vi "Query Multi Eval Meas Spectrum Limit Check Results.vi"(0 "VISA resource name":refnum<visa-resource-name>, 5 "Instance (1)":i32=1, 7 "Result Type (Current)":i32(ring) items=["Current"=0, "Maximum"=4], 11 "error in (no error)":errorcluster) -> (4 "VISA resource name out":refnum<visa-resource-name>, 6 "Reliability":i32, 8 "Limit Check Results":dbl[](array[numeric]), 14 "Out Of Tolerance":i32, 15 "error out":errorcluster)   [LabVIEW 2020, in "Rohde&Schwarz CMP LR WPAN Measurement.lvlib"]
doc: "Returns the spectrum limit check single results.\n\nAttribute:\n-\n\nRemote-control commands:\nCALCulate:WPAN:MEAS<i>:MEValuation:SPECtrum:CURRent?\nCALCulate:WPAN:MEAS<i>:MEValuation:SPECtrum:MAXimum?"
uses:
  <instrlib>/Rohde&Schwarz CMP LR WPAN Measurement/Rohde&Schwarz CMP LR WPAN Measurement.lvlib
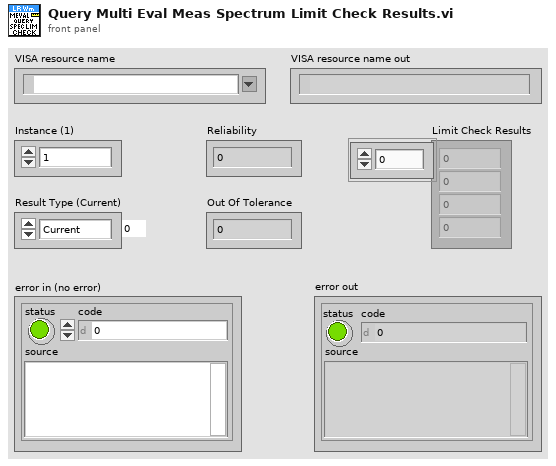
[diagram p1: front panel]
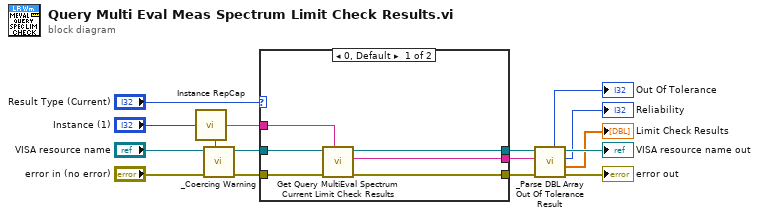
[diagram p0: block diagram]
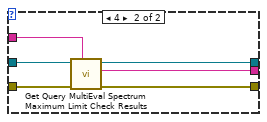
[diagram p2: hidden frame]
diagram:
  n1 = call <instrlib>:"Instance RepCap.vi"("Instance In"="Instance (1)") -> ("In Range?"=w15:bool, "RepCap Identifier Out"=w16:string)  [unwired: 1 in]
  n2 = call <instrlib>:"_Coercing Warning.vi"("In Range?"=w15, "error in (no error)"="error in (no error)", "VISA resource name"="VISA resource name") -> ("error out"=w12:errorcluster, "VISA resource name out"=w11:refnum<visa-resource-name>)  [unwired: 7 in]
  n3 = case shown="0, Default" "Result Type (Current)" {
    tunnel: w16 -> [w22 w28]
    tunnel: w11 -> [w20 w26]
    tunnel: w12 -> [w21 w27]
    tunnel: [w19 w25] -> w9
    tunnel: [w18 w24] -> w4
    tunnel: [w17 w23] -> w3
    frame 0, Default {
      n4 = call "Get Query MultiEval Spectrum Current Limit Check Results"("Repeated Capabilities"=w22, "error in (no error)"=w21, "instrument handle"=w20) -> ("error out"=w18:errorcluster, "Query MultiEval Spectrum Current Limit Check Results"=w17:string, "instrument handle out"=w19:refnum<visa-resource-name>)  [unwired: 6 in]
    }
    frame 4 {
      n5 = call "Get Query MultiEval Spectrum Maximum Limit Check Results"("Repeated Capabilities"=w28, "error in (no error)"=w27, "instrument handle"=w26) -> ("error out"=w24:errorcluster, "Query MultiEval Spectrum Maximum Limit Check Results"=w23:string, "instrument handle out"=w25:refnum<visa-resource-name>)  [unwired: 6 in]
    }
  }
  n6 = call <instrlib>:"_Parse DBL Array Out Of Tolerance Result.vi"("error in (no error)"=w4, "Input String"=w3, "VISA resource name"=w9) -> ("error out"=→"error out":errorcluster, "Results"=→"Limit Check Results":dbl[], "Reliability"=→"Reliability":i32, "VISA resource name out"=→"VISA resource name out":refnum<visa-resource-name>, "Out Of Tolerance"=→"Out Of Tolerance":i32)  [unwired: 4 in]
